vi "Teleop.vi"(10 "Match Info":T2={"Autonomous Elapsed Seconds"=0.0, "TeleOp Elapsed Seconds"=0.0, "Disabled Elapsed Seconds"=0.0, "Visited Autonomous"=FALSE, "Visited TeleOp"=FALSE, "Visited Disabled"=FALSE, "Autonomous Settings"={"Autonomous Style"=enum."Independent", "VI Refnum"=refnum}}, 11 "Call Context":T3) -> ()   [LabVIEW 2011]
doc: "This VI is called for each TeleOp packet received from the DS where the robot is not disabled. It is often used to read from the joysticks and update I/O or to update setpoints for timed control loops. It should complete and return within 20 milliseconds or it may miss DS packets."
uses:
  <vilib>/Rock Robotics/WPI/DriverStation/WPI_DriverStationDerivedRobotMode.ctl
  <vilib>/Rock Robotics/WPI/DriverStation/WPI_DriverStationMatch Info.ctl
  <vilib>/Rock Robotics/WPI/Solenoid/WPI_SolenoidValue.ctl
  Robot Global Data.vi
  <vilib>/Rock Robotics/WPI/Solenoid/WPI_SolenoidSetEnum.vi
  <vilib>/Rock Robotics/WPI/Solenoid/Deprecated/WPI_SolenoidGetBool.vi
  <vilib>/Rock Robotics/WPI/Compressor/WPI_CompressorGetSetRefNum.vi
panel:
  out "Sonar Distance Average":dbl
  out "Sonar Distance Output":dbl
  out "Battery Voltage":dbl
  out "Sonar Voltage":dbl
  in  "Value":T1
  out "Shift":bool
  out "Enabled?":bool
  in  "Accel Rate":dbl=0.1
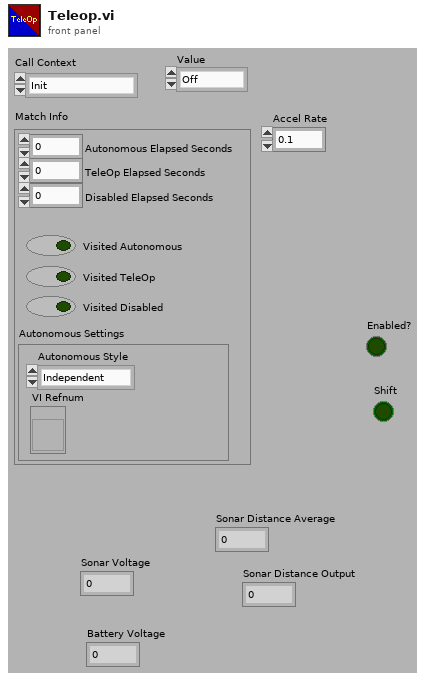
[diagram p1: front panel]
types:
  T1 = typedef "WPI_SolenoidValue.ctl" = enum16{"Off", "On", "Forward", "Reverse"}
  T2 = typedef "WPI_DriverStationMatch Info.ctl" = cluster{"Autonomous Elapsed Seconds":dbl, "TeleOp Elapsed Seconds":dbl, "Disabled Elapsed Seconds":dbl, "Visited Autonomous":bool, "Visited TeleOp":bool, "Visited Disabled":bool, "Autonomous Settings":cluster{"Autonomous Style":enum16{"Iterative", "Independent"}, "VI Refnum":refnum<vi>}}
  T3 = typedef "WPI_DriverStationDerivedRobotMode.ctl" = enum16{"Init", "Execute", "Stop"}
  T4 = typedef "WPI_JoystickDevRef.ctl" = cluster{"Device":T5}
  T5 = typedef "WPI_JoystickDeviceEnum.ctl" = enum16{"USB 1", "USB 2", "USB 3", "USB 4", "Kinect 1", "Kinect 2"}
  T6 = typedef "WPI_JoystickButtonState.ctl" = cluster{"Button 1":bool, "Button 2":bool, "Button 3":bool, "Button 4":bool, "Button 5":bool, "Button 6":bool, "Button 7":bool, "Button 8":bool, "Button 9":bool, "Button 10":bool, "Button 11":bool, "Button 12":bool}
  T7 = cluster{"axis 1 (x)":dbl, "axis 2 (y)":dbl, "axis 3 (throttle)":dbl, "axis 4":dbl, "axis 5":dbl, "axis 6":dbl}
  T8 = typedef "WPI_SolenoidDevRef.ctl" = cluster{"DevStatus":errorcluster, "Solenoid Module":T9, "Forward Solenoid Channel":T10, "Reverse Solenoid Channel":T10}
  T9 = typedef "FPGA_TypedefSolenoidModule.ctl" = enum16{"Solenoid Module 1", "Solenoid Module 2"}
  T10 = typedef "WPI_SolenoidChannel.ctl" = enum8{"Solenoid 1", "Solenoid 2", "Solenoid 3", "Solenoid 4", "Solenoid 5", "Solenoid 6", "Solenoid 7", "Solenoid 8", "Invalid"}
  T11 = typedef "WPI_CompressorDevRef.ctl" = cluster{"DevStatus":errorcluster, "DigitalInputDevRef":T12, "RelayDevRef":T15}
  T12 = typedef "WPI_DigitalInputDevRef.ctl" = cluster{"DevStatus":errorcluster, "DIO Channel":T13, "Digital Module":T14}
  T13 = typedef "FPGA_DIOChannel.ctl" = enum8{"DIO 1", "DIO 2", "DIO 3", "DIO 4", "DIO 5", "DIO 6", "DIO 7", "DIO 8", "DIO 9", "DIO 10", "DIO 11", "DIO 12", "DIO 13", "DIO 14", "Invalid"}
  T14 = typedef "FPGA_TypedefDigitalModule.ctl" = enum16{"Digital Module 1", "Digital Module 2"}
  T15 = typedef "WPI_RelayDevRef.ctl" = cluster{"DevStatus":errorcluster, "Relay Channel":T16, "Digital Module":T14, "Relay Direction":T17}
  T16 = typedef "FPGA_DIORelayChannel.ctl" = enum8{"Relay 1", "Relay 2", "Relay 3", "Relay 4", "Relay 5", "Relay 6", "Relay 7", "Relay 8", "Invalid"}
  T17 = typedef "WPI_RelayDirection.ctl" = enum16{"Both directions", "Forward only", "Reverse only"}
  T18 = typedef "WPI_AnalogChannelDevRef.ctl" = cluster{"DevStatus":errorcluster, "Analog Module":T19, "Analog Channel":T20}
  T19 = typedef "FPGA_TypedefAnalogModule.ctl" = enum16{"Analog Module 1", "Analog Module 2"}
  T20 = typedef "FPGA_AIChannel.ctl" = enum8{"AI 1", "AI 2", "AI 3", "AI 4", "AI 5", "AI 6", "AI 7", "AI 8", "Invalid"}
  T21 = typedef "WPI_RobotDriveDevRef.ctl" = cluster{"DevStatus":errorcluster, "Motors[]":T22[], "Square Inputs":bool, "Max Output":dbl, "Isochronous":bool}
  T22 = typedef "WPI_MotorControlDeviceRef.ctl" = cluster{"DeviceStatus":errorcluster, "Type":enum16{"PWM", "CAN"}, "PWM":cluster{"Digital Module":T14, "PWM Channel":T23, "DeadBand":T24}, "CAN":cluster{"Device Number":u8, "Control Mode":T25, "Semaphore":T26, "Max Vout":dbl}, "Invert":bool, "TransformRef":T27, "InvTransformRef":T27}
  T23 = typedef "FPGA_DIOPWMChannel.ctl" = enum8{"PWM 1", "PWM 2", "PWM 3", "PWM 4", "PWM 5", "PWM 6", "PWM 7", "PWM 8", "PWM 9", "PWM 10", "Invalid"}
  T24 = typedef "WPI_PWMDeadband.ctl" = cluster{"Name":string, "maxPositivePwm":i32, "minPositivePwm":i32, "centerPwm":i32, "maxNegativePwm":i32, "minNegativePwm":i32, "angularRange":u16}
  T25 = typedef "WPI_CANJaguar_ControlMode.ctl" = enum8{"Percent VBus", "Current", "Speed", "Position", "Voltage"}
  T26 = typedef "Semaphore RefNum" = refnum<k1>
  T27 = typedef "WPI_PWMTransform_ConPane.ctl" = refnum<vi>
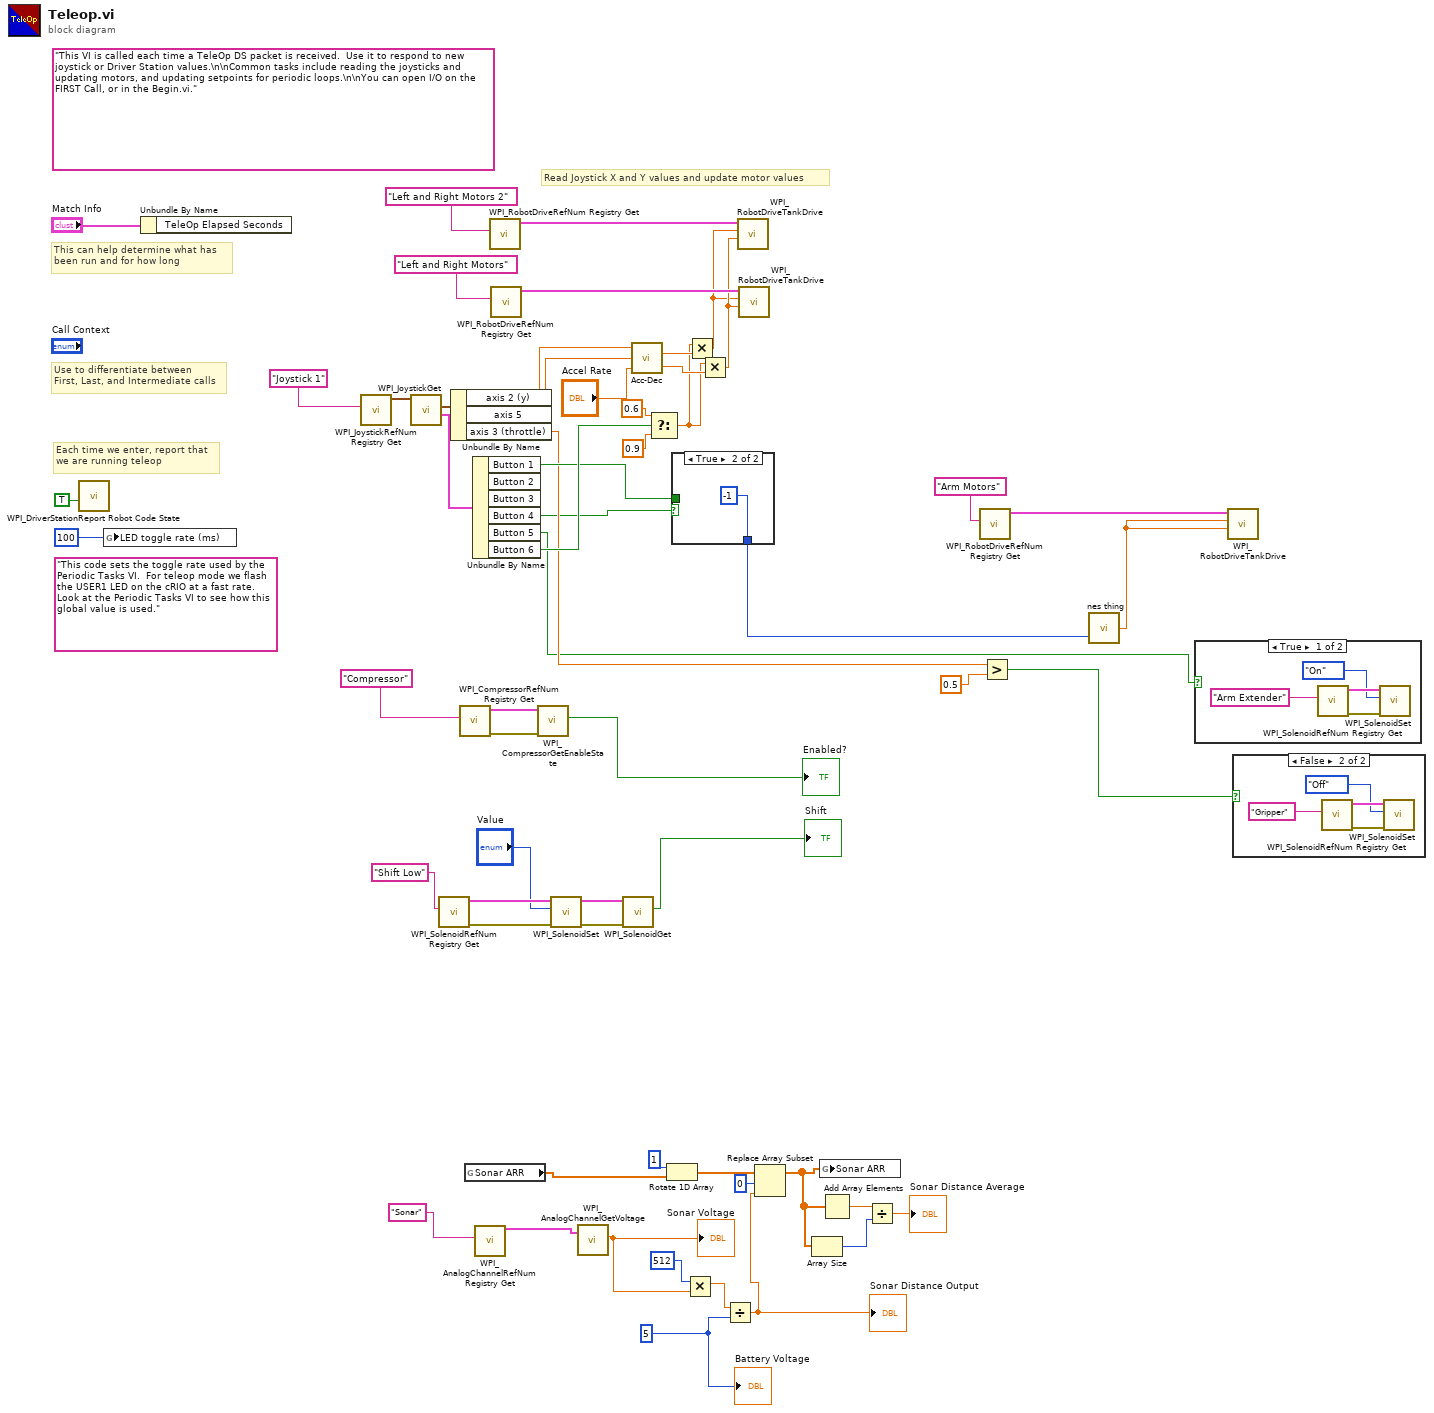
[diagram p0: block diagram]
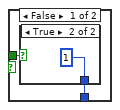
[diagram p2: hidden frame]
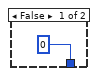
[diagram p3: hidden frame]
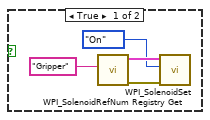
[diagram p4: hidden frame]
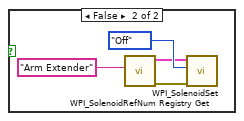
[diagram p5: hidden frame]
diagram:
  w29 = 5
  (unwired) "This code sets the toggle rate used by the Periodic Tasks VI.  For teleop mode we flash the USER1 LED on the cRIO at a fast rate.  Look at the Periodic Tasks VI to see how this global value is used."
  (unwired) "This VI is called each time a TeleOp DS packet is received.  Use it to respond to new joystick or Driver Station values.\n\nCommon tasks include reading the joysticks and updating motors, and updating setpoints for periodic loops.\n\nYou can open I/O on the FIRST Call, or in the Begin.vi."
  # "Each time we enter, report that\nwe are running teleop"
  # "Use to differentiate between\nFirst, Last, and Intermediate calls"
  # "This can help determine what has\nbeen run and for how long"
  # "Read Joystick X and Y values and update motor values"
  n1 = call <vilib>:"WPI_DriverStationReport Robot Code State.vi"("TeleOp"=TRUE ("Autonomous")) -> ()  [unwired: 10 in, 1 out]
  n2 = global write "Robot Global Data.vi" "LED toggle rate (ms)"(u32 100 ("LED ms toggle rate")) -> ()
  n3 = Unbundle By Name("Match Info") -> ()  [unwired: 1 out]
  n4 = call <vilib>:"WPI_JoystickRefNum Registry Get.vi"("refnum name"="Joystick 1") -> ("JoystickDevRef"=w53:T4)  [unwired: 1 in, 9 out]
  n5 = call <vilib>:"WPI_JoystickGet.vi"("JoystickDevRef"=w53) -> ("Buttons"=w12:T6, "Axes"=w55:T7)  [unwired: 1 in, 4 out]
  n6 = call <vilib>:"WPI_SolenoidRefNum Registry Get.vi"("refnum name"="Shift Low") -> ("error out"=w38:errorcluster, "SolenoidDevRef"=w37:T8)  [unwired: 9 in]
  n7 = Unbundle By Name(w55) -> ("axis 2 (y)"=w14:dbl, "axis 5"=w13:dbl, "axis 3 (throttle)"=w4:dbl)
  n8 = call <vilib>:"WPI_CompressorRefNum Registry Get.vi"("refnum name"="Compressor") -> ("error out"=w40:errorcluster, "CompressorDevRef"=w43:T11)  [unwired: 9 in]
  n9 = global read "Robot Global Data.vi" "Sonar ARR"() -> (w26:dbl[])
  n10 = Unbundle By Name(w12) -> ("Button 1"=w7:bool, "Button 4"=w1:bool, "Button 5"=w2:bool, "Button 6"=w8:bool)  [unwired: 2 out]
  n11 = call <vilib>:"WPI_AnalogChannelRefNum Registry Get.vi"("refnum name"="Sonar") -> ("AIDeviceRef"=w28:T18)  [unwired: 9 in, 1 out]
  n12 = call <vilib>:"WPI_RobotDriveRefNum Registry Get.vi"("refnum name"="Left and Right Motors 2") -> ("RobotDriveDevRef"=w48:T21)  [unwired: 1 in, 9 out]
  n13 = call <vilib>:"WPI_RobotDriveRefNum Registry Get.vi"("refnum name"="Left and Right Motors") -> ("RobotDriveDevRef"=w56:T21)  [unwired: 1 in, 9 out]
  n14 = call <vilib>:"WPI_CompressorGetEnableState.vi"("error in (no error)"=w40, "CompressorDevRef"=w43) -> ("Enabled"=→"Enabled?":bool)  [unwired: 6 in, 3 out]
  n15 = call-poly <vilib>:"WPI_SolenoidSet.vi"("error in (no error)"=w38, "Value"="Value", "SolenoidDevRef"=w37) -> ("error out"=w34:errorcluster, "SolenoidDevRef"=w35:T8)  [unwired: 7 in]
  n16 = call <vilib>:"WPI_AnalogChannelGetVoltage.vi"("AIDeviceRef"=w28) -> ("Voltage"=w27:dbl)  [unwired: 8 in, 2 out]
  "Sonar Voltage" <- w27
  n17 = call-poly <vilib>:"WPI_SolenoidGet.vi"("error in (no error)"=w34, "SolenoidDevRef"=w35) -> ("Value"=→"Shift":bool)  [unwired: 7 in, 2 out]
  n18 = call "Acc-Dec.vi"("Acc Rate"="Accel Rate", "Y-Input 2"=w13, "Y-Input 1"=w14) -> ("Y-Output 2"=w47:dbl, "Y-Output 1"=w15:dbl)
  n19 = Select(t=0.6, s=w8, f=0.9) -> (s? t:f=w10:dbl)
  n20 = Rotate 1D Array(1:w26, 2:1) -> (0:w24:dbl[])
  n21 = case shown="True" w1 {
    tunnel: w7 -> [w60 _]
    tunnel: [w59 -1] -> w6
    frame False {
      n22 = case shown="True" w60 {
        tunnel: [0 1] -> w59
        frame False {
        }
        frame True {
        }
      }
    }
    frame True {
    }
  }
  n23 = Multiply(x=512, y=w27) -> (x*y=w30:dbl)
  n24 = Multiply(x=w10, y=w15) -> (x*y=w16:dbl)
  n25 = Multiply(x=w10, y=w47) -> (x*y=w17:dbl)
  n26 = Divide(x=w30, y=w29) -> (x/y=w23:dbl)
  "Sonar Distance Output" <- w23
  n27 = call <vilib>:"WPI_RobotDriveTankDrive.vi"("Right axis value"=w17, "Left axis value"=w16, "RobotDriveDevRef"=w48) -> ()  [unwired: 7 in, 2 out]
  n28 = call <vilib>:"WPI_RobotDriveTankDrive.vi"("Right axis value"=w17, "Left axis value"=w16, "RobotDriveDevRef"=w56) -> ()  [unwired: 7 in, 2 out]
  n29 = Replace Array Subset(array=w24, new element=w23, index=0) -> (w20:dbl[])
  n30 = Array Size(array=w20) -> (size(s)=w19:i32)
  n31 = global write "Robot Global Data.vi" "Sonar ARR"(w20) -> ()
  n32 = Add Array Elements(numeric array=w20) -> (sum=w21:dbl)
  n33 = Divide(x=w21, y=w19) -> (x/y=→"Sonar Distance Average":dbl)
  n34 = call <vilib>:"WPI_RobotDriveRefNum Registry Get.vi"("refnum name"="Arm Motors") -> ("RobotDriveDevRef"=w45:T21)  [unwired: 1 in, 9 out]
  n35 = Greater?(x=w4, y=0.5) -> (0:w3:bool)
  n36 = call "nes thing.vi"("Y- Axis"=w6) -> ("Powah"=w44:dbl)  [unwired: 1 in]
  n37 = case shown="True" w2 {
    frame True {
      n38 = call <vilib>:"WPI_SolenoidRefNum Registry Get.vi"("refnum name"="Arm Extender") -> ("error out"=w66:errorcluster, "SolenoidDevRef"=w65:T8)  [unwired: 9 in]
      n39 = call-poly <vilib>:"WPI_SolenoidSet.vi"("error in (no error)"=w66, "Value"=WPI_SolenoidValue."On", "SolenoidDevRef"=w65) -> ()  [unwired: 7 in, 2 out]
    }
    frame False {
      n40 = call <vilib>:"WPI_SolenoidRefNum Registry Get.vi"("refnum name"="Arm Extender") -> ("error out"=w69:errorcluster, "SolenoidDevRef"=w70:T8)  [unwired: 9 in]
      n41 = call-poly <vilib>:"WPI_SolenoidSet.vi"("error in (no error)"=w69, "Value"=WPI_SolenoidValue."Off", "SolenoidDevRef"=w70) -> ()  [unwired: 7 in, 2 out]
    }
  }
  n42 = call <vilib>:"WPI_RobotDriveTankDrive.vi"("Right axis value"=w44, "Left axis value"=w44, "RobotDriveDevRef"=w45) -> ()  [unwired: 7 in, 2 out]
  n43 = case shown="False" w3 {
    frame True {
      n44 = call <vilib>:"WPI_SolenoidRefNum Registry Get.vi"("refnum name"="Gripper") -> ("error out"=w75:errorcluster, "SolenoidDevRef"=w74:T8)  [unwired: 9 in]
      n45 = call-poly <vilib>:"WPI_SolenoidSet.vi"("error in (no error)"=w75, "Value"=WPI_SolenoidValue."On", "SolenoidDevRef"=w74) -> ()  [unwired: 7 in, 2 out]
    }
    frame False {
      n46 = call <vilib>:"WPI_SolenoidRefNum Registry Get.vi"("refnum name"="Gripper") -> ("error out"=w78:errorcluster, "SolenoidDevRef"=w77:T8)  [unwired: 9 in]
      n47 = call-poly <vilib>:"WPI_SolenoidSet.vi"("error in (no error)"=w78, "Value"=WPI_SolenoidValue."Off", "SolenoidDevRef"=w77) -> ()  [unwired: 7 in, 2 out]
    }
  }
  "Battery Voltage" <- w29
